vi "Compile Engine Init.vi"(8 "error in (no error)":errorcluster, 11 "Device Item Ref in":T2 format="%.0x") -> (0 "error out":errorcluster, 2 "System":T1, 3 "Device Item Ref out":T2 format="%.0x")   [LabVIEW 2013, in "Engine Simulation Toolkit System Explorer.lvlib"]
uses:
  Engine Simulation Toolkit System Explorer.lvlib
  <vilib>/NI Veristand/Custom Device API/Custom Device Item Ref.ctl
  Shared/Engine Init Data.ctl
  <vilib>/NI Veristand/Custom Device API/Custom Device Channel Type.ctl
  Shared/Properties.vi
  <vilib>/NI Veristand/Custom Device API/Get Item Property (I32).vi
  <vilib>/NI Veristand/Custom Device API/Get Item Property (String).vi
  <vilib>/NI Veristand/Custom Device API/Get Item Property (Boolean).vi
  <vilib>/NI Veristand/Custom Device API/Get Item Property (Dependent File).vi
  Shared/Engine Simulation Toolkit Shared.lvlib
  <vilib>/NI Veristand/Custom Device API/Custom Device API.lvlib
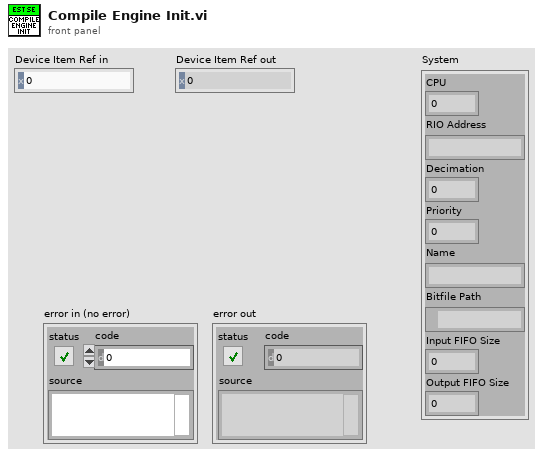
[diagram p1: front panel]
types:
  T1 = typedef "Engine Simulation Toolkit Shared.lvlib/Engine Init Data.ctl" = cluster{"CPU":i32, "RIO Address":string, "Decimation":i64, "Priority":i32, "Name":string, "Bitfile Path":path, "Input FIFO Size":i32, "Output FIFO Size":i32}
  T2 = typedef "Custom Device API.lvlib/Custom Device Item Ref.ctl" = u64
  T3 = typedef "Custom Device API.lvlib/Custom Device Channel Type.ctl" = enum16{"Input", "Output"}
  T4 = typedef "Custom Device API.lvlib/Custom Device Timed Loop Priority.ctl" = enum32{"Low", "Medium", "High"}
  T5 = typedef "Custom Device API.lvlib/Custom Device Item Info.ctl" = cluster{"Name":string, "Is Channel":bool, "GUID":string, "Is Waveform":bool}
  T6 = typedef "Custom Device API.lvlib/Custom Device Target Type.ctl" = enum16{"PharLap", "VxWorks", "Windows"}
  T7 = typedef "Custom Device API.lvlib/Dependent File Optional Info.ctl" = cluster{"Version":string, "RTDestination":path, "ForceDownload":bool, "SupportedTarget":string, "MD5":string}
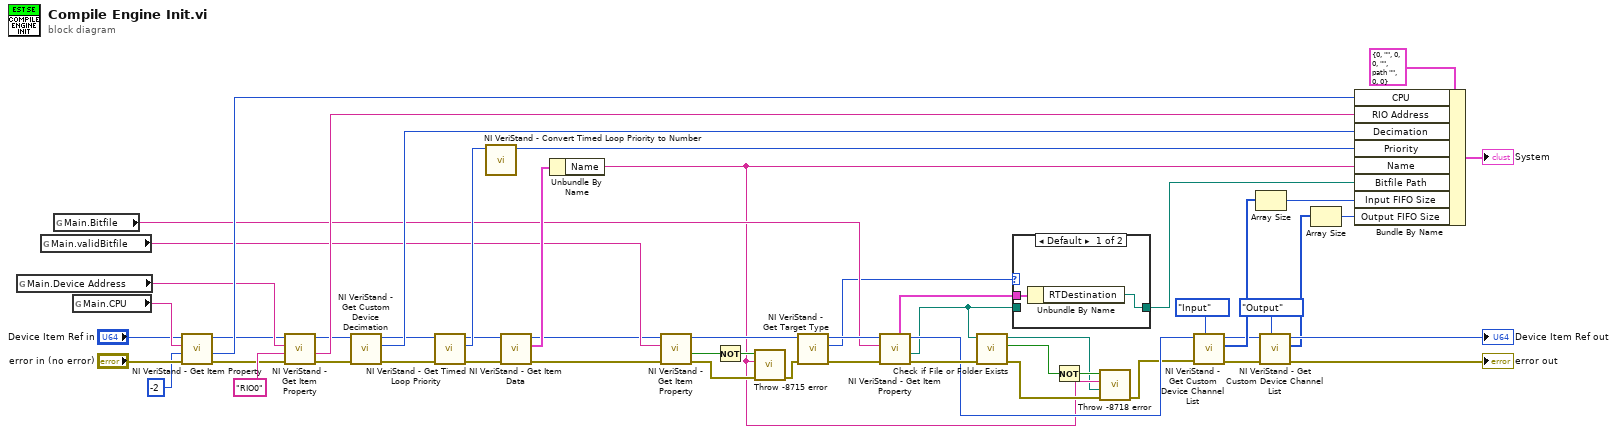
[diagram p0: block diagram]
diagram:
  n1 = global read "Properties.vi" "Main.Device Address"() -> (w49:string)
  n2 = global read "Properties.vi" "Main.validBitfile"() -> (w30:string)
  n3 = global read "Properties.vi" "Main.Bitfile"() -> (w26:string)
  n4 = global read "Properties.vi" "Main.CPU"() -> (w53:string)
  n5 = call-poly <vilib>:"NI VeriStand - Get Item Property.vi"("error in (no error)"="error in (no error)", "Default Value"=-2, "Property Name"=w53, "Item Ref in"="Device Item Ref in") -> ("error out"=w47:errorcluster, "Value"=w51:i32, "Item Ref out"=w48:T2)  [unwired: 4 in, 1 out]
  n6 = call-poly <vilib>:"NI VeriStand - Get Item Property.vi"("error in (no error)"=w47, "Default Value"="RIO0", "Property Name"=w49, "Item Ref in"=w48) -> ("error out"=w46:errorcluster, "Value"=w45:string, "Item Ref out"=w43:T2)  [unwired: 4 in, 1 out]
  n7 = call <vilib>:"NI VeriStand - Get Custom Device Decimation.vi"("error in (no error)"=w46, "Device Ref in"=w43) -> ("error out"=w44:errorcluster, "Decimation"=w42:i32, "Device Ref out"=w40:T2)  [unwired: 7 in]
  n8 = call <vilib>:"NI VeriStand - Get Timed Loop Priority.vi"("error in (no error)"=w44, "Device Ref in"=w40) -> ("error out"=w41:errorcluster, "Priority"=w39:T4, "Device Ref out"=w37:T2)  [unwired: 7 in]
  n9 = call <vilib>:"NI VeriStand - Convert Timed Loop Priority to Number.vi"("Priority"=w39) -> ("Numeric Priority"=w38:i32)  [unwired: 10 in]
  n10 = call <vilib>:"NI VeriStand - Get Item Data.vi"("error in (no error)"=w41, "Item Ref in"=w37) -> ("error out"=w21:errorcluster, "Item Info"=w36:T5, "Item Ref out"=w20:T2)  [unwired: 6 in, 1 out]
  n11 = Unbundle By Name(w36) -> ("Name"=w2:string)
  n12 = call-poly <vilib>:"NI VeriStand - Get Item Property.vi"("error in (no error)"=w21, "Property Name"=w30, "Item Ref in"=w20) -> ("error out"=w28:errorcluster, "Value"=w29:bool, "Item Ref out"=w31:T2)  [unwired: 5 in, 1 out]
  n13 = Not(x=w29) -> (.not. x?=w9:bool)
  n14 = call "Throw -8715 error.vi"("error in (no error)"=w28, "Custom device name"=w2, "Error"=w9) -> ("error out"=w27:errorcluster)  [unwired: 8 in]
  n15 = call <vilib>:"NI VeriStand - Get Target Type.vi"("error in (no error)"=w27, "Item Ref in"=w31) -> ("error out"=w35:errorcluster, "Target Type"=w25:T6, "Item Ref out"=w33:T2)  [unwired: 7 in]
  n16 = call-poly <vilib>:"NI VeriStand - Get Item Property.vi"("error in (no error)"=w35, "Property Name"=w26, "Item Ref in"=w33) -> ("error out"=w34:errorcluster, "Path"=w7:path, "Item Ref out"=w8:T2, "OptionalInfo"=w24:T7)  [unwired: 4 in, 1 out]
  n17 = call <vilib>:"Check if File or Folder Exists.vi"("error in (no error)"=w34, "path"=w7) -> ("error out"=w6:errorcluster, "file or folder exists?"=w4:bool, "dup path"=w1:path)  [unwired: 7 in]
  n18 = case shown="Default" w25 {
    tunnel: w24 -> [w57 _]
    tunnel: w7 -> [_ w58]
    tunnel: [w56 w58] -> w23
    frame Default {
      n19 = Unbundle By Name(w57) -> ("RTDestination"=w56:path)
    }
    frame "Windows" {
    }
  }
  n20 = Not(x=w4) -> (.not. x?=w3:bool)
  n21 = call "Throw -8718 error.vi"("error in (no error)"=w6, "path"=w1, "Custom device name"=w2, "Error"=w3) -> ("error out"=w5:errorcluster)  [unwired: 7 in]
  n22 = call <vilib>:"NI VeriStand - Get Custom Device Channel List.vi"("Channel Type"=Custom_Device_Channel_Type."Input", "error in (no error)"=w5, "Device Ref in"=w8) -> ("error out"=w19:errorcluster, "Specified Channel Ref List"=w17:T2[], "Device Ref out"=w14:T2)  [unwired: 6 in]
  n23 = Array Size(array=w17) -> (size(s)=w16:i32)
  n24 = call <vilib>:"NI VeriStand - Get Custom Device Channel List.vi"("Channel Type"=Custom_Device_Channel_Type."Output", "error in (no error)"=w19, "Device Ref in"=w14) -> ("error out"=→"error out":errorcluster, "Specified Channel Ref List"=w11:T2[], "Device Ref out"=→"Device Item Ref out":T2)  [unwired: 6 in]
  n25 = Array Size(array=w11) -> (size(s)=w10:i32)
  n26 = Bundle By Name(cluster=T1 {"CPU"=0, "RIO Address"="", "Decimation"=0, "Priority"=0, "Name"="", "Bitfile Path"=path "", "Input FIFO Size"=0, "Output FIFO Size"=0} ("System"), "CPU"=w51, "RIO Address"=w45, "Decimation"=w42, "Priority"=w38, "Name"=w2, "Bitfile Path"=w23, "Input FIFO Size"=w16, "Output FIFO Size"=w10) -> (→"System":T1)
